vi "AddTestSuite.vi"(8 "error in (no error)":errorcluster, 10 "TestSuite":refnum<class "TestSuite.lvclass">, 11 "TestSuite in":refnum<class "TestSuite.lvclass">) -> (0 "error out":errorcluster, 3 "TestSuite out":refnum<class "TestSuite.lvclass">)   [LabVIEW 2019, in "TestSuite.lvclass"]
doc: "Adds a test suite."
uses:
  TestSuite.lvclass
  C:/Users/de200256/Code/LVUnit/Test/Test.lvclass
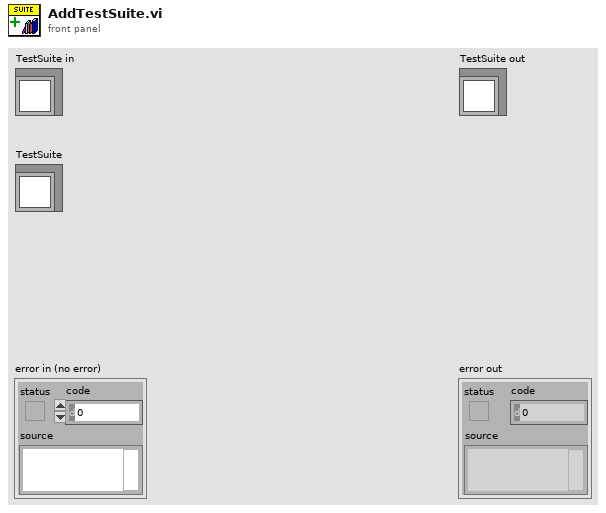
[diagram p1: front panel]
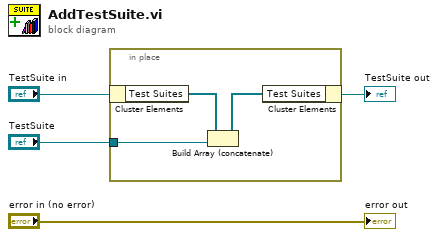
[diagram p0: block diagram]
diagram:
  n1 = in-place {
    in-place-border: "TestSuite" -> [w6]
    n2 = in-place-cluster #1("TestSuite in") -> ("Test Suites"=w7:refnum<class "Test.lvclass">[])
    n3 = Build Array (concatenate)(w7, w6) -> (w5:refnum<class "Test.lvclass">[])
    n4 = in-place-cluster #1("Test Suites"=w5) -> (→"TestSuite out":refnum<class "TestSuite.lvclass">)
  }
  "error out" <- "error in (no error)"
